vi "Global names.vi"() -> ()   [LabVIEW 2015]
panel:
  out "LOG exit":string="LOG module closed"
  out "LOG initialized":string="LOG module initialized"
  out "DAQ exit":string="DAQ module closed"
  out "DAQ updated":string="DAQ channels updated"
  out "DAQ initialized":string="DAQ module initialized"
  out "Model exit":string="Model closed"
  out "Barrel filled":string="Another barrel filled"
  out "Overflow":string="Liquid level overflow!"
  out "Model initialized":string="Model initilalized"
  out "Line unpowered":string="No power!"
  out "Line powered":string="Line has been powered"
  out "Started":string="Process has started"
  out "PLC initializing":string="Initializing PLC..."
  out "PLC init successful":string="PLC initialization successful!"
  out "PLC closing":string="Closing PLC..."
  out "PLC shutdown":string="PLC shutdown successful!"
  out "Stopped":string="Process has stoped"
  out "Stopping":string="Stopping process..."
  out "Starting":string="Starting process..."
  in  "Status log dir":string="data"
  # "Application statuses"
  # "Exit statuses"
  # "Open statuses"
  # "Other statuses"
  # "Folder names"
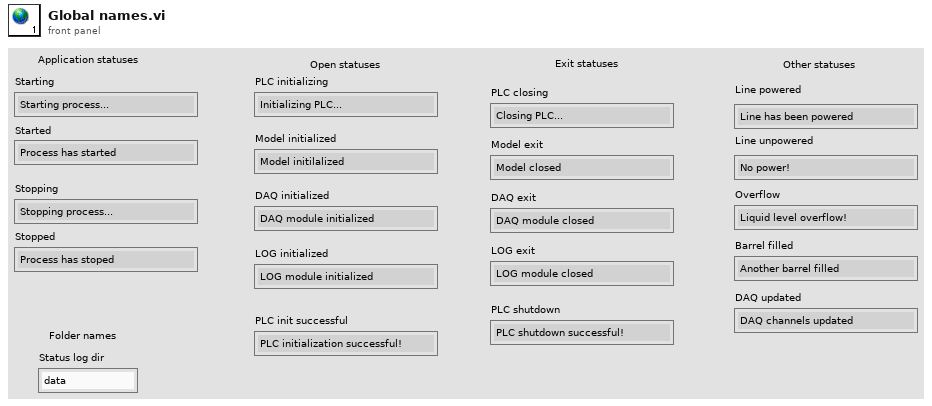
[diagram p1: front panel]
diagram:
